vi "Execute Command (No results).vi"(8 "error in (no error)":errorcluster, 9 "Parameters":variant, 10 "SQL":string, 11 "PQ Connection in":refnum<class "PQ Connection.lvclass">) -> (0 "error out":errorcluster, 3 "PQ Connection out":refnum<class "PQ Connection.lvclass">)   [LabVIEW 2013, in "PQ Connection.lvclass"]
doc: "Execute one or more SQL commands. Optionally, one can provide parameters to be bound to $n tokens in the SQL command (eg. \"SELECT * FROM mytable WHERE x = $1\"). If parameters are provided than only one SQL command can be executed. The parameters can be a cluster or an array, or can be a single value if only one parameter is needed."
uses:
  PQ Connection.lvclass
  Result/PQ Result.lvclass
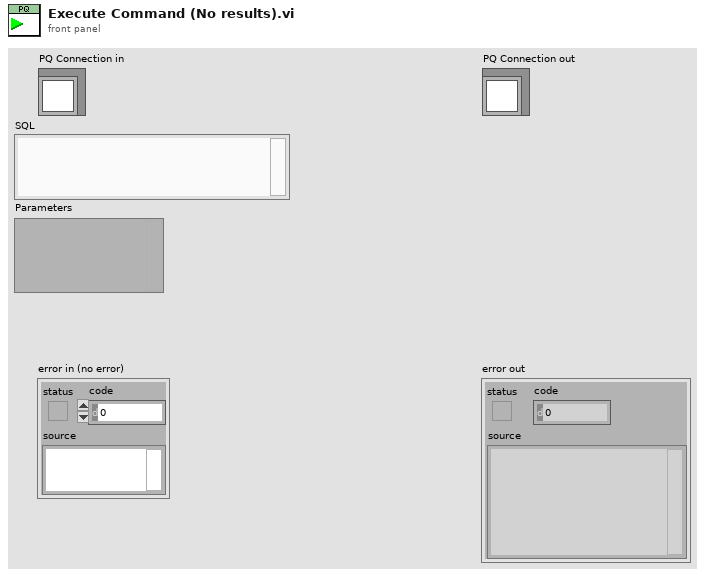
[diagram p1: front panel]
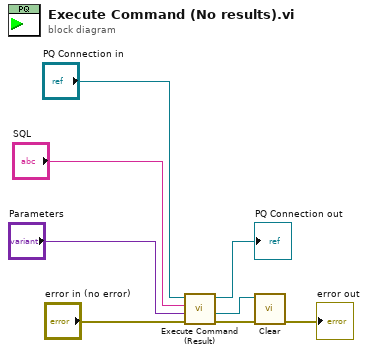
[diagram p0: block diagram]
diagram:
  n1 = call "Execute Command (Result).vi"("error in (no error)"="error in (no error)", "Parameter(s)"="Parameters", "SQL"="SQL", "PQ Connection in"="PQ Connection in") -> ("error out"=w4:errorcluster, "First Result with Rows returned"=w6:refnum<class "PQ Result.lvclass">, "PQ Connection out"=→"PQ Connection out":refnum<class "PQ Connection.lvclass">)  [unwired: 4 in, 1 out]
  n2 = call "Clear.vi"("error in (no error)"=w4, "PQ Result  in"=w6) -> ("error out"=→"error out":errorcluster)  [unwired: 9 in]
